vi "DefenderPenalty.vi"(6 "N atacantes":u32[](array[numeric]), 10 "Total de n \natacantes":i32, 11 "Robot in":T1) -> (3 "Robot out":T1)   [LabVIEW 2016]
uses:
  Core/AI Robot.ctl
  Functions Enum.ctl
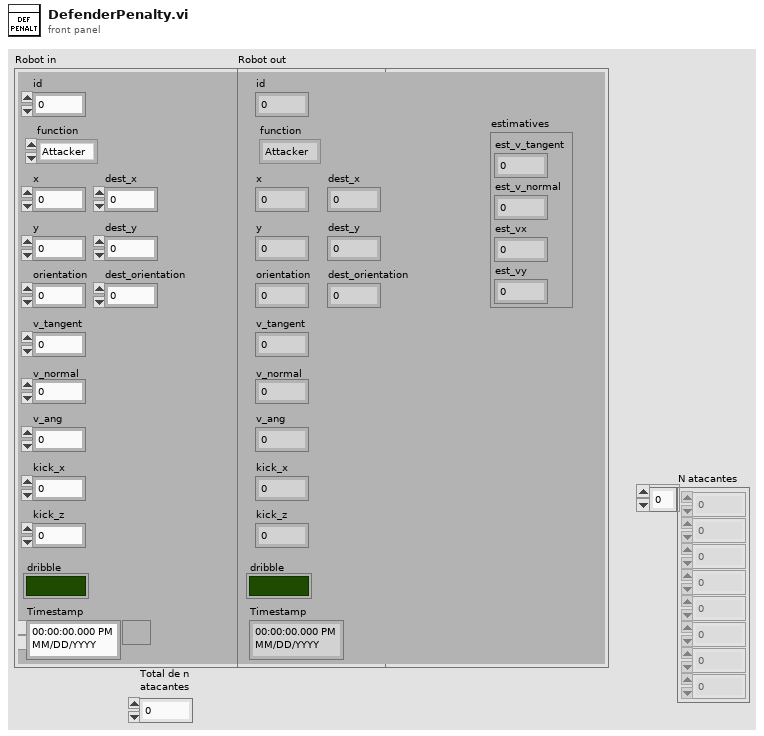
[diagram p1: front panel]
types:
  T1 = typedef "AI Robot.ctl" = cluster{"id":u32, "function":T2, "x":dbl, "y":dbl, "orientation":dbl, "v_tangent":dbl, "v_normal":dbl, "v_ang":dbl, "kick_x":dbl, "kick_z":dbl, "dribble":bool, "Timestamp":timestamp, "dest_x":dbl, "dest_y":dbl, "dest_orientation":dbl, "estimatives":cluster{"est_v_tangent":dbl, "est_v_normal":dbl, "est_vx":dbl, "est_vy":dbl}}
  T2 = typedef "Functions Enum.ctl" = enum16{"Attacker", "Goalie", "Defender", "Striker", "Goto 0", "Dummy", "ZigZag"}
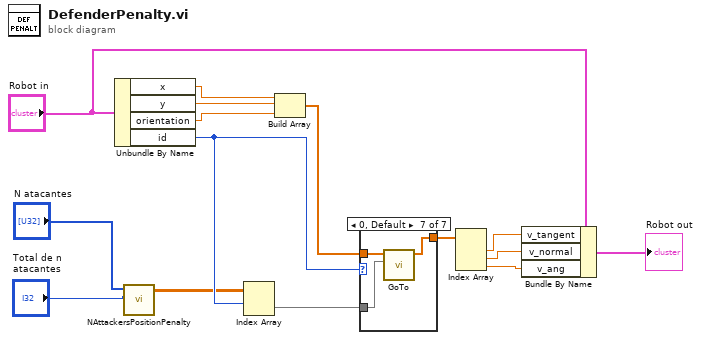
[diagram p0: block diagram]
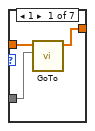
[diagram p2: hidden frame]
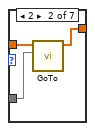
[diagram p3: hidden frame]
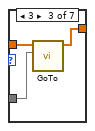
[diagram p4: hidden frame]
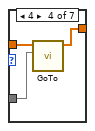
[diagram p5: hidden frame]
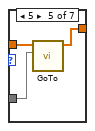
[diagram p6: hidden frame]
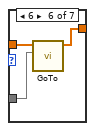
[diagram p7: hidden frame]
diagram:
  n1 = Unbundle By Name("Robot in") -> ("x"=w15:dbl, "y"=w14:dbl, "orientation"=w13:dbl, "id"=w5:u32)
  n2 = call "NAttackersPositionPenalty.vi"("N atacantes"="N atacantes", "Total de n \natacantes"="Total de n \natacantes") -> ("Posição dos não atacantes\ndurante o penalte"=w3:dbl[][])  [unwired: 8 in]
  n3 = Index Array(array=w3, index (row)=w5) -> (element=w4:dbl[])  [unwired: 1 in]
  n4 = Build Array(w15, w14, w13) -> (w12:dbl[])
  n5 = case shown="0, Default" w5 {
    tunnel: w12 -> [w18 w21 w24 w27 w30 w33 w36]
    tunnel: [w17 w20 w23 w26 w29 w32 w35] -> w11
    tunnel: w4 -> [w16 w19 w22 w25 w28 w31 w34]
    frame 1 {
      n6 = call "GoTo.vi"("Target"=w16, "Position"=w18) -> ("Output\nVelocity"=w17:dbl[])  [unwired: 8 in, 1 out]
    }
    frame 2 {
      n7 = call "GoTo.vi"("Target"=w19, "Position"=w21) -> ("Output\nVelocity"=w20:dbl[])  [unwired: 8 in, 1 out]
    }
    frame 3 {
      n8 = call "GoTo.vi"("Target"=w22, "Position"=w24) -> ("Output\nVelocity"=w23:dbl[])  [unwired: 8 in, 1 out]
    }
    frame 4 {
      n9 = call "GoTo.vi"("Target"=w25, "Position"=w27) -> ("Output\nVelocity"=w26:dbl[])  [unwired: 8 in, 1 out]
    }
    frame 5 {
      n10 = call "GoTo.vi"("Target"=w28, "Position"=w30) -> ("Output\nVelocity"=w29:dbl[])  [unwired: 8 in, 1 out]
    }
    frame 6 {
      n11 = call "GoTo.vi"("Target"=w31, "Position"=w33) -> ("Output\nVelocity"=w32:dbl[])  [unwired: 8 in, 1 out]
    }
    frame 0, Default {
      n12 = call "GoTo.vi"("Target"=w34, "Position"=w36) -> ("Output\nVelocity"=w35:dbl[])  [unwired: 8 in, 1 out]
    }
  }
  n13 = Index Array(array=w11) -> (element #1=w9:dbl, element #2=w8:dbl, element #3=w7:dbl)  [unwired: 3 in]
  n14 = Bundle By Name(cluster="Robot in", "v_tangent"=w9, "v_normal"=w8, "v_ang"=w7) -> (→"Robot out":T1)
